vi "escritura.vi"() -> ()   [LabVIEW 2020]
panel:
  out "Waveform Chart":dynamicdata(graph)
  in  "TEMPERATURA":dbl(slide) scale=0.0..100.0
  in  "DETENER":bool
  out "ALARMA":bool
  in  "LIMITE":dbl
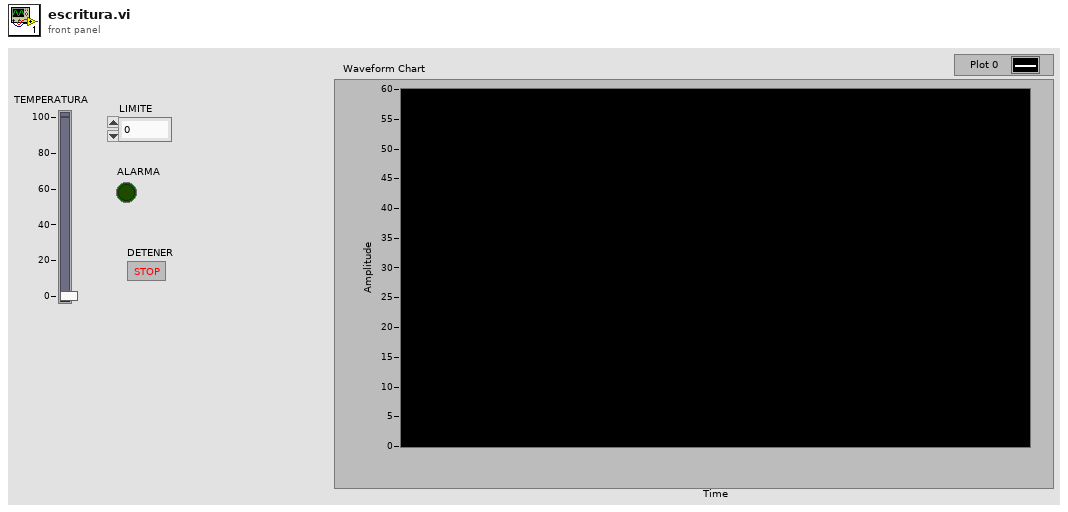
[diagram p1: front panel]
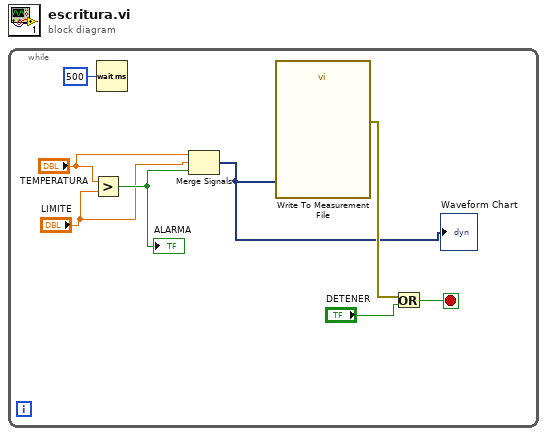
[diagram p0: block diagram]
diagram:
  n1 = while {
    stop <- w2 stop-if-true
    n2 = Greater?(x="TEMPERATURA", y="LIMITE") -> (0:w7:bool)
    "ALARMA" <- w7
    n3 = Wait (ms)(milliseconds to wait=u32 500) -> ()  [unwired: 1 out]
    n4 = Merge Signals("TEMPERATURA", "LIMITE", w7) -> (w1:dynamicdata)
    "Waveform Chart" <- w1
    n5 = call "Write To Measurement File"("Signals"=w1) -> ("error out"=w4:errorcluster)  [unwired: 16 in, 2 out]
    n6 = Or(x=w4, y="DETENER") -> (x .or. y?=w2:bool)
  }
